vi "Destroy.vi"(0 "reference in":refnum<class "SPWB.lvclass">, 5 "error in (no error)":errorcluster) -> (14 "reference out":refnum<class "SPWB.lvclass">, 19 "error out":errorcluster)   [LabVIEW 2022 SP3, in "SPWB.lvclass"]
doc: "Destructor."
uses:
  SPWB.lvclass
  API/Generic Utilities_class/Generic Utilities.lvclass
  API/Registration_class/Registration.lvclass
  API/GSwFormDSP_class/GSwFormDSP.lvclass
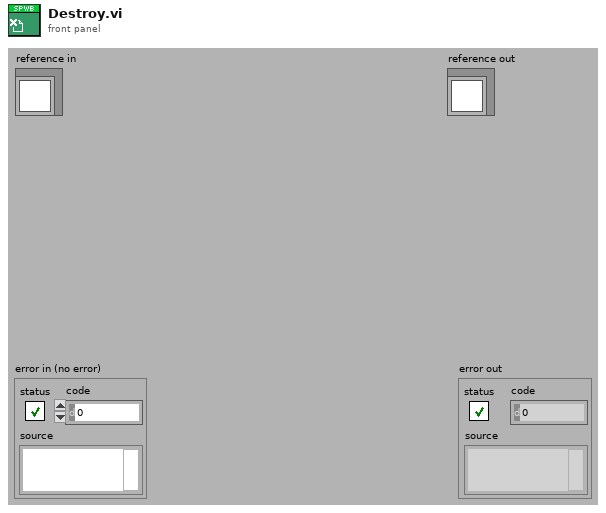
[diagram p1: front panel]
types:
  T1 = typedef "SPWB.lvclass/ObjectAttributes.ctl" = cluster{"Window Name Index":string, "Data":refnum<class "GSwFormDSP.lvclass">, "Registration":refnum<class "Registration.lvclass">, "TFA User Control Refs ":T2}
  T2 = typedef "SPWB.lvclass/TFA - User Control References.ctl" = cluster{"STFT Graph":refnum<vi>, "Time Section":refnum<vi>, "Frequency Section":refnum<vi>}
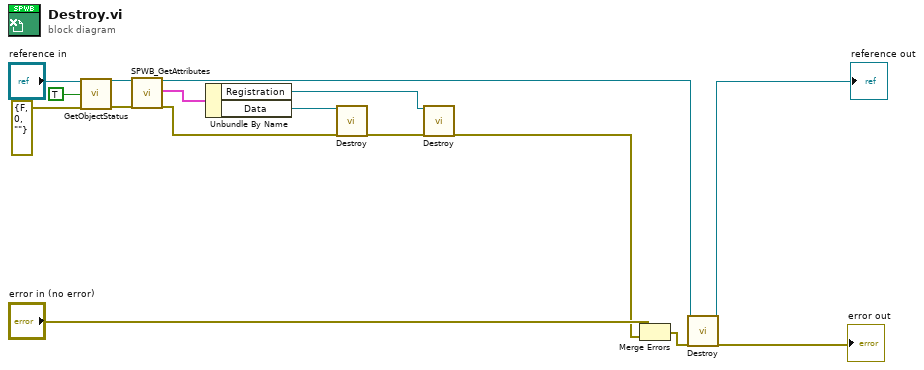
[diagram p0: block diagram]
diagram:
  n1 = call-dynamic "GetObjectStatus.vi"("reference in"="reference in", "simple info (F)"=TRUE ("simple info"), "error in (no error)"=errorcluster {"status"=FALSE, "code"=0, "source"=""}) -> ("reference out"=w10:refnum<class "SPWB.lvclass">, "error out"=w11:errorcluster)  [unwired: 5 in, 10 out]
  n2 = call "SPWB_GetAttributes.vi"("reference in"=w10, "error in (no error)"=w11) -> ("reference out"=w9:refnum<class "SPWB.lvclass">, "attributes"=w8:T1, "error out"=w4:errorcluster)  [unwired: 14 in, 1 out]
  n3 = Unbundle By Name(w8) -> ("Registration"=w1:refnum<class "Registration.lvclass">, "Data"=w5:refnum<class "GSwFormDSP.lvclass">)
  n4 = call-dynamic "Destroy.vi"("reference in"=w5, "error in (no error)"=w4) -> ("error out"=w3:errorcluster)  [unwired: 16 in, 1 out]
  n5 = call-dynamic "Destroy.vi"("reference in"=w1, "error in (no error)"=w3) -> ("error out"=w2:errorcluster)  [unwired: 16 in, 1 out]
  n6 = Merge Errors("error in (no error)", w2) -> (w15:errorcluster)
  n7 = call-parent "Destroy.vi"("reference in"=w9, "error in (no error)"=w15) -> ("reference out"=→"reference out":refnum<class "SPWB.lvclass">, "error out"=→"error out":errorcluster)  [unwired: 16 in]
